vi "ex06_array.vi"() -> ()   [LabVIEW 2019]
panel:
  in  "Switches":bool[](array[boolean])
  out "Tanks":dbl[](array[slide]) scale=0.0..10.0
  out "LEDs":bool[](array[boolean])
  out "Meters":dbl[](array[knob]) scale=0.0..10.0
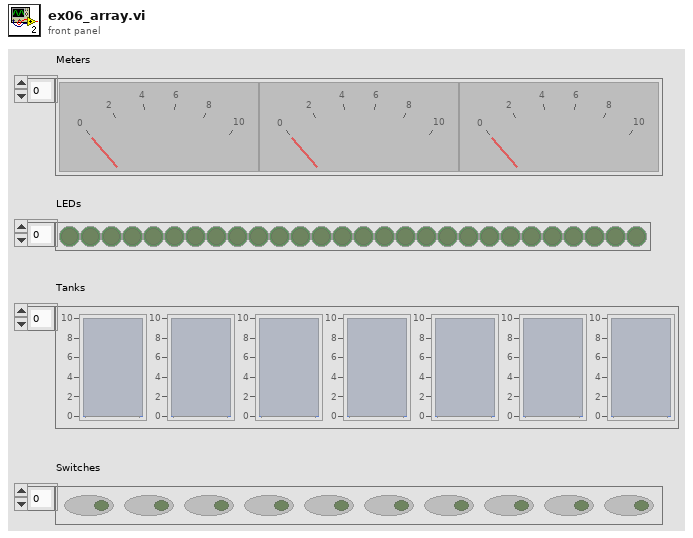
[diagram p1: front panel]
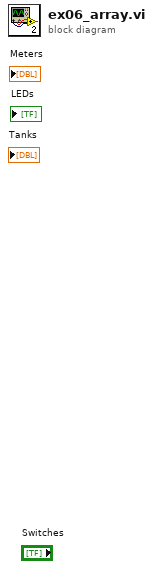
[diagram p0: block diagram]
diagram:
